vi "TrafficLight.vi"() -> ()   [LabVIEW 2020]
panel:
  in  "Car Speed":dbl(slide) scale=10.0..200.0
  out "E_3":bool
  out "E_2":bool
  out "E_1":bool
  out "W_3":bool
  out "W_2":bool
  out "W_1":bool
  out "S_3":bool
  out "S_2":bool
  out "S_1":bool
  out "N_3":bool
  out "N_2":bool
  out "N_1":bool
  in  "START":bool
  in  "EMERGENCY":bool
  in  "EW_Green Light Duration":dbl(slide) scale=5.0..30.0
  in  "NS_Green Light Duration":dbl(slide) scale=5.0..30.0
  in  "stop":bool
  out "W_R":bool
  out "W_Y":bool
  out "W_G":bool
  out "E_G":bool
  out "E_Y":bool
  out "E_R":bool
  out "S_G":bool
  out "S_Y":bool
  out "S_R":bool
  out "N_R":bool
  out "N_Y":bool
  out "N_G":bool
  # "Simulation Interface"
  # "Control Panel"
  # "North"
  # "West"
  # "East"
  # "South"
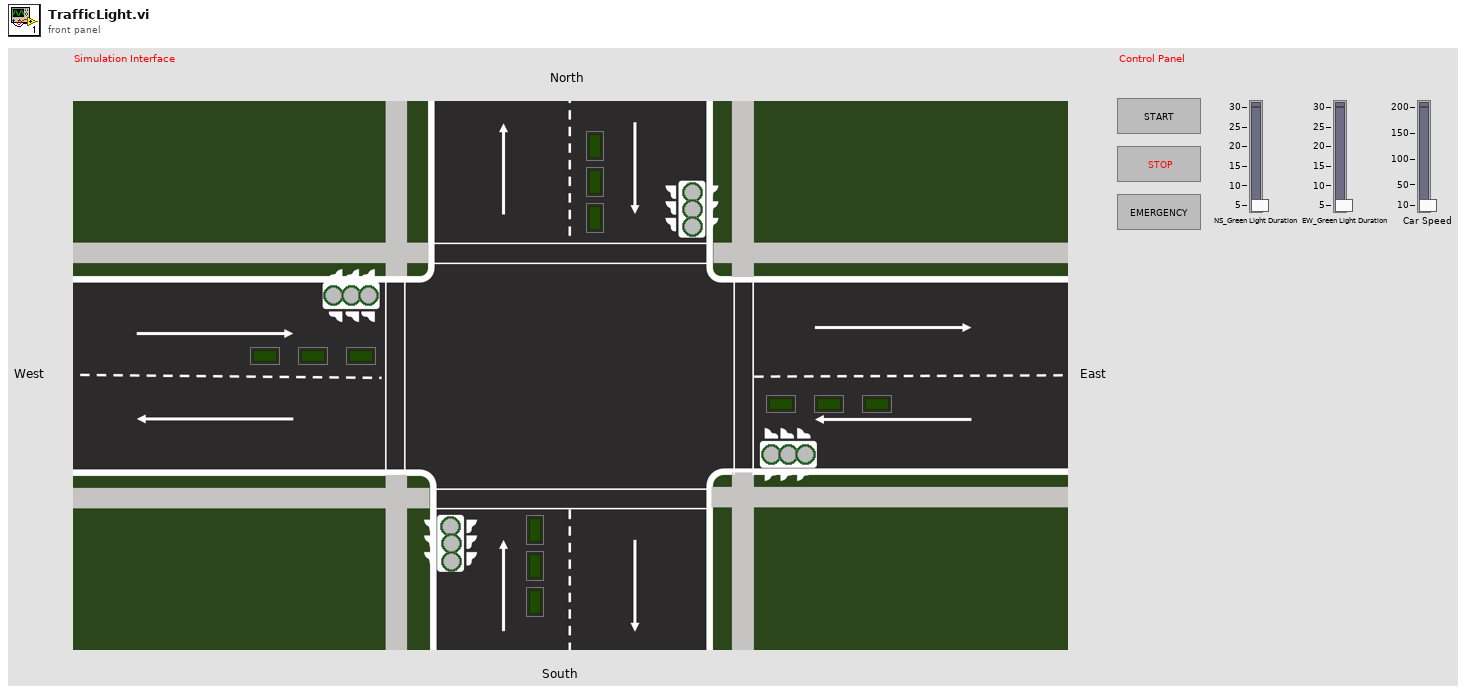
[diagram p1: front panel]
types:
  T1 = enum16{"Start", "Green", "Yellow", "Red", "Yellow'"}
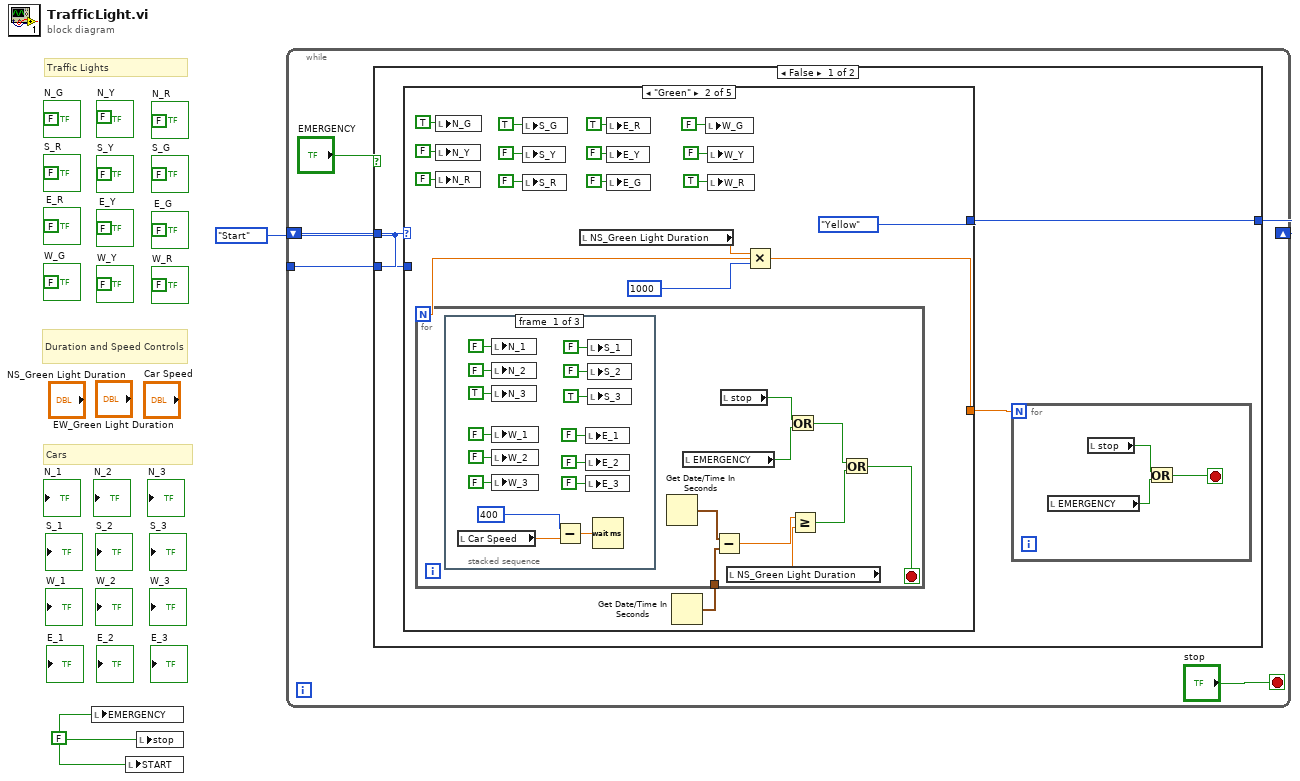
[diagram p0: block diagram]
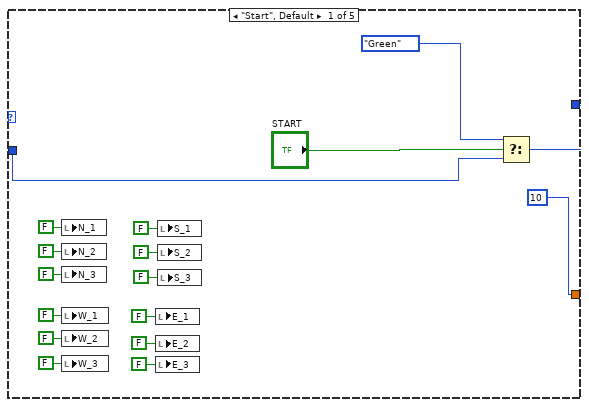
[diagram p2: hidden frame]
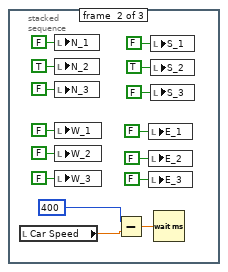
[diagram p3: hidden frame]
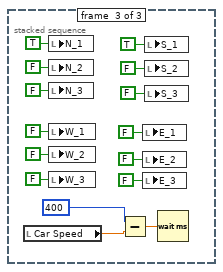
[diagram p4: hidden frame]
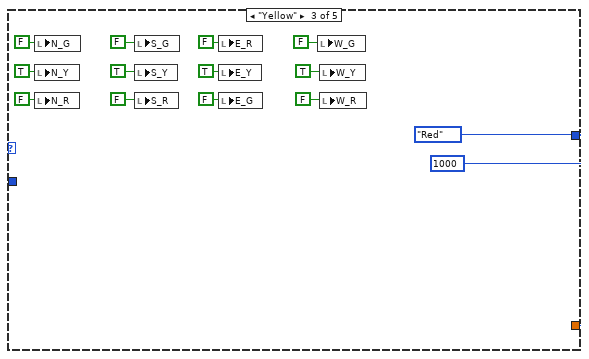
[diagram p5: hidden frame]
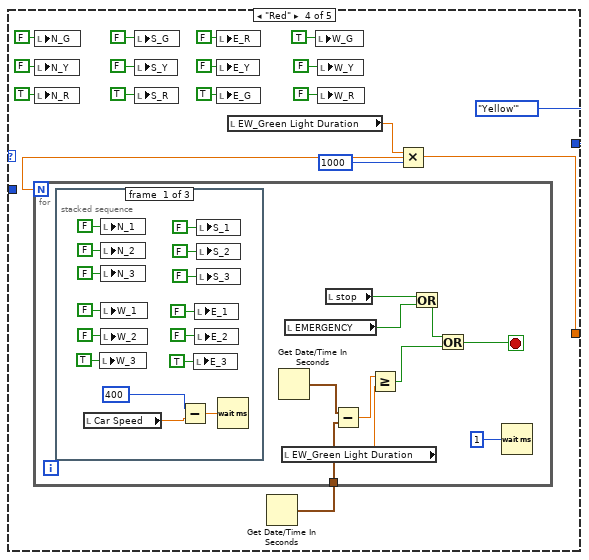
[diagram p6: hidden frame]
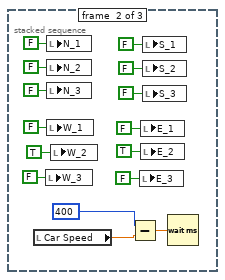
[diagram p7: hidden frame]
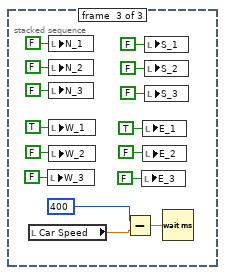
[diagram p8: hidden frame]
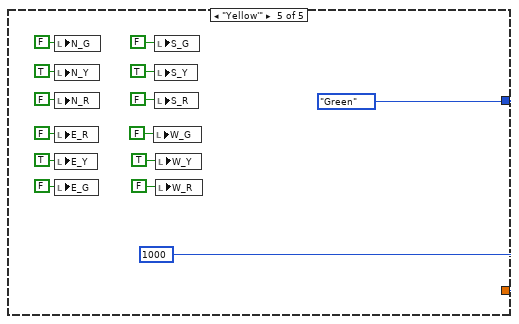
[diagram p9: hidden frame]
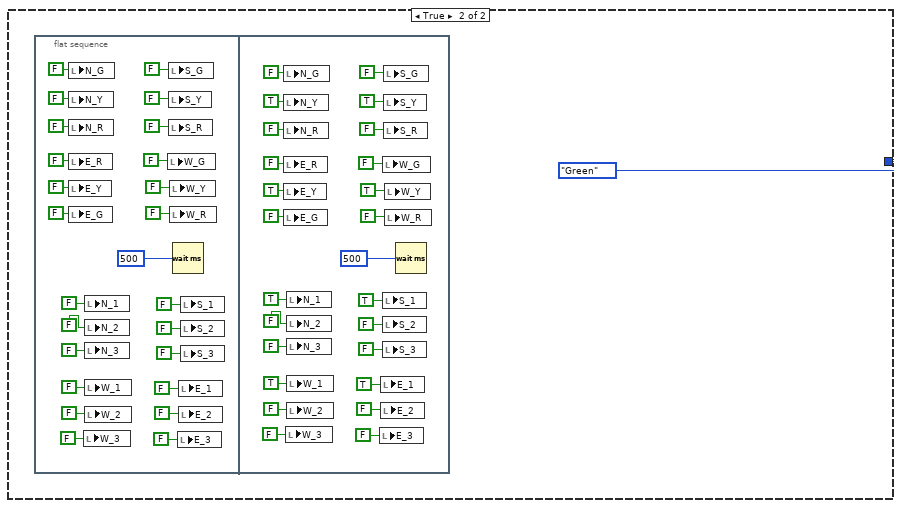
[diagram p10: hidden frame]
diagram:
  w1 = FALSE ("EMERGENCY")
  w2 = T1."Start"
  # "Cars"
  # "Duration and Speed Controls"
  # "Traffic Lights"
  n1 = local write "EMERGENCY"(w1) -> ()
  n2 = local write "START"(w1) -> ()
  n3 = local write "stop"(w1) -> ()
  n4 = while {
    shift-right: [w15] -> _
    shift-left: w2 -> [w17]
    tunnel: w2 -> [w16]
    stop <- "stop" stop-if-true
    n5 = case shown="False" "EMERGENCY" {
      tunnel: w17 -> [w23 _]
      tunnel: w16 -> [w22 _]
      tunnel: [w21 T1."Green"] -> w15
      frame False {
        n6 = case shown="\"Green\"" w23 {
          tunnel: w22 -> [w42 _ _ _ _]
          tunnel: [w40 T1."Yellow" T1."Red" T1."Yellow'" T1."Green"] -> w21
          tunnel: [10 w53 u32 1000 ("millisecond timer value") w130 u32 1000 ("millisecond timer value")] -> w20
          frame "Start", Default {
            (unwired) FALSE ("W_2")
            n7 = local write "N_1"(FALSE ("N_1")) -> ()
            n8 = local write "N_2"(FALSE ("N_2")) -> ()
            n9 = local write "N_3"(FALSE ("N_3")) -> ()
            n10 = local write "W_1"(FALSE ("W_1")) -> ()
            n11 = local write "W_2"(FALSE ("W_2")) -> ()
            n12 = local write "W_3"(FALSE ("W_3")) -> ()
            n13 = local write "E_1"(FALSE ("E_1")) -> ()
            n14 = local write "E_2"(FALSE ("E_2")) -> ()
            n15 = local write "E_3"(FALSE ("E_3")) -> ()
            n16 = local write "S_1"(FALSE ("S_1")) -> ()
            n17 = local write "S_2"(FALSE ("S_2")) -> ()
            n18 = local write "S_3"(FALSE ("S_3")) -> ()
            n19 = Select(t=T1."Green", s="START", f=w42) -> (s? t:f=w40:T1)
          }
          frame "Green" {
            n20 = local write "N_G"(TRUE ("N_G")) -> ()
            n21 = local write "N_Y"(FALSE ("N_Y")) -> ()
            n22 = local write "N_R"(FALSE ("N_R")) -> ()
            n23 = local write "S_G"(TRUE ("S_G")) -> ()
            n24 = local write "S_Y"(FALSE ("S_Y")) -> ()
            n25 = local write "S_R"(FALSE ("E_R")) -> ()
            n26 = local read "NS_Green Light Duration"() -> (w56:dbl)
            n27 = local write "E_R"(TRUE ("E_R")) -> ()
            n28 = local write "E_Y"(FALSE ("E_Y")) -> ()
            n29 = local write "E_G"(FALSE ("E_G")) -> ()
            n30 = Get Date/Time In Seconds() -> (seconds since 1Jan1904=w54:timestamp)
            n31 = local write "W_G"(FALSE ("W_G")) -> ()
            n32 = local write "W_Y"(FALSE ("W_Y")) -> ()
            n33 = local write "W_R"(TRUE ("W_R")) -> ()
            n34 = Multiply(x=w56, y=u32 1000 ("millisecond timer value")) -> (x*y=w53:dbl)
            n35 = for {
              N: w53 -> [_]
              tunnel: w54 -> [w68]
              stop <- w64 stop-if-true
              n36 = stacked-sequence {
                frame #0 {
                  (unwired) FALSE ("W_2")
                  n37 = local read "Car Speed"() -> (w70:dbl)
                  n38 = local write "N_1"(FALSE ("N_1")) -> ()
                  n39 = local write "N_2"(FALSE ("N_2")) -> ()
                  n40 = local write "N_3"(TRUE ("N_3")) -> ()
                  n41 = local write "W_1"(FALSE ("W_1")) -> ()
                  n42 = local write "W_2"(FALSE ("W_2")) -> ()
                  n43 = local write "W_3"(FALSE ("W_3")) -> ()
                  n44 = Subtract(x=u32 400 ("millisecond timer value"), y=w70) -> (x-y=w72:dbl)
                  n45 = local write "E_1"(FALSE ("E_1")) -> ()
                  n46 = local write "E_2"(FALSE ("E_2")) -> ()
                  n47 = local write "E_3"(FALSE ("E_3")) -> ()
                  n48 = local write "S_1"(FALSE ("S_1")) -> ()
                  n49 = local write "S_2"(FALSE ("S_2")) -> ()
                  n50 = local write "S_3"(TRUE ("S_3")) -> ()
                  n51 = Wait (ms)(milliseconds to wait=w72) -> ()  [unwired: 1 out]
                }
                frame #1 {
                  (unwired) FALSE ("W_2")
                  n52 = local read "Car Speed"() -> (w87:dbl)
                  n53 = local write "N_1"(FALSE ("N_1")) -> ()
                  n54 = local write "N_2"(TRUE ("N_2")) -> ()
                  n55 = local write "N_3"(FALSE ("N_3")) -> ()
                  n56 = local write "W_1"(FALSE ("W_1")) -> ()
                  n57 = local write "W_2"(FALSE ("W_2")) -> ()
                  n58 = local write "W_3"(FALSE ("W_3")) -> ()
                  n59 = Subtract(x=u32 400 ("millisecond timer value"), y=w87) -> (x-y=w85:dbl)
                  n60 = local write "E_1"(FALSE ("E_1")) -> ()
                  n61 = local write "E_2"(FALSE ("E_2")) -> ()
                  n62 = local write "E_3"(FALSE ("E_3")) -> ()
                  n63 = local write "S_1"(FALSE ("S_1")) -> ()
                  n64 = local write "S_2"(TRUE ("S_2")) -> ()
                  n65 = local write "S_3"(FALSE ("S_3")) -> ()
                  n66 = Wait (ms)(milliseconds to wait=w85) -> ()  [unwired: 1 out]
                }
                frame #2 {
                  (unwired) FALSE ("W_2")
                  n67 = local read "Car Speed"() -> (w100:dbl)
                  n68 = local write "N_1"(TRUE ("N_1")) -> ()
                  n69 = local write "N_2"(FALSE ("N_2")) -> ()
                  n70 = local write "N_3"(FALSE ("N_3")) -> ()
                  n71 = local write "W_1"(FALSE ("W_1")) -> ()
                  n72 = local write "W_2"(FALSE ("W_2")) -> ()
                  n73 = local write "W_3"(FALSE ("W_3")) -> ()
                  n74 = Subtract(x=u32 400 ("millisecond timer value"), y=w100) -> (x-y=w102:dbl)
                  n75 = local write "E_1"(FALSE ("E_1")) -> ()
                  n76 = local write "E_2"(FALSE ("E_2")) -> ()
                  n77 = local write "E_3"(FALSE ("E_3")) -> ()
                  n78 = local write "S_1"(TRUE ("S_1")) -> ()
                  n79 = local write "S_2"(FALSE ("S_2")) -> ()
                  n80 = local write "S_3"(FALSE ("S_3")) -> ()
                  n81 = Wait (ms)(milliseconds to wait=w102) -> ()  [unwired: 1 out]
                }
              }
              n82 = Get Date/Time In Seconds() -> (seconds since 1Jan1904=w69:timestamp)
              n83 = local read "EMERGENCY"() -> (w62:bool)
              n84 = Subtract(x=w69, y=w68) -> (x-y=w67:dbl)
              n85 = local read "stop"() -> (w63:bool)
              n86 = local read "NS_Green Light Duration"() -> (w66:dbl)
              n87 = Or(x=w63, y=w62) -> (x .or. y?=w61:bool)
              n88 = Greater Or Equal?(x=w67, y=w66) -> (x >= y?=w65:bool)
              n89 = Or(x=w61, y=w65) -> (x .or. y?=w64:bool)
            }
          }
          frame "Yellow" {
            n90 = local write "N_G"(FALSE ("N_G")) -> ()
            n91 = local write "N_Y"(TRUE ("N_Y")) -> ()
            n92 = local write "N_R"(FALSE ("N_R")) -> ()
            n93 = local write "S_G"(FALSE ("S_G")) -> ()
            n94 = local write "S_Y"(TRUE ("S_Y")) -> ()
            n95 = local write "S_R"(FALSE ("E_R")) -> ()
            n96 = local write "E_R"(FALSE ("E_R")) -> ()
            n97 = local write "E_Y"(TRUE ("E_Y")) -> ()
            n98 = local write "E_G"(FALSE ("E_G")) -> ()
            n99 = local write "W_G"(FALSE ("W_G")) -> ()
            n100 = local write "W_Y"(TRUE ("W_Y")) -> ()
            n101 = local write "W_R"(FALSE ("W_R")) -> ()
          }
          frame "Red" {
            n102 = local write "N_G"(FALSE ("N_G")) -> ()
            n103 = local write "N_Y"(FALSE ("N_Y")) -> ()
            n104 = local write "N_R"(TRUE ("N_R")) -> ()
            n105 = local write "S_G"(FALSE ("S_G")) -> ()
            n106 = local write "S_Y"(FALSE ("S_Y")) -> ()
            n107 = local write "S_R"(TRUE ("E_R")) -> ()
            n108 = local write "E_R"(FALSE ("E_R")) -> ()
            n109 = local write "E_Y"(FALSE ("E_Y")) -> ()
            n110 = local write "E_G"(TRUE ("E_G")) -> ()
            n111 = local read "EW_Green Light Duration"() -> (w131:dbl)
            n112 = Get Date/Time In Seconds() -> (seconds since 1Jan1904=w129:timestamp)
            n113 = local write "W_G"(TRUE ("W_G")) -> ()
            n114 = local write "W_Y"(FALSE ("W_Y")) -> ()
            n115 = local write "W_R"(FALSE ("W_R")) -> ()
            n116 = Multiply(x=w131, y=1000) -> (x*y=w130:dbl)
            n117 = for {
              N: w130 -> [_]
              tunnel: w129 -> [w153]
              stop <- w146 stop-if-true
              n118 = stacked-sequence {
                frame #0 {
                  (unwired) FALSE ("W_2")
                  n119 = local read "Car Speed"() -> (w156:dbl)
                  n120 = local write "W_3"(TRUE ("W_3")) -> ()
                  n121 = local write "N_1"(FALSE ("N_1")) -> ()
                  n122 = local write "N_2"(FALSE ("N_2")) -> ()
                  n123 = local write "N_3"(FALSE ("N_3")) -> ()
                  n124 = local write "W_1"(FALSE ("W_1")) -> ()
                  n125 = local write "W_2"(FALSE ("W_2")) -> ()
                  n126 = Subtract(x=u32 400 ("millisecond timer value"), y=w156) -> (x-y=w158:dbl)
                  n127 = local write "E_3"(TRUE ("E_3")) -> ()
                  n128 = local write "E_1"(FALSE ("E_1")) -> ()
                  n129 = local write "E_2"(FALSE ("E_2")) -> ()
                  n130 = local write "S_1"(FALSE ("S_1")) -> ()
                  n131 = local write "S_2"(FALSE ("S_2")) -> ()
                  n132 = local write "S_3"(FALSE ("S_3")) -> ()
                  n133 = Wait (ms)(milliseconds to wait=w158) -> ()  [unwired: 1 out]
                }
                frame #1 {
                  n134 = local read "Car Speed"() -> (w175:dbl)
                  n135 = local write "W_3"(FALSE ("W_3")) -> ()
                  n136 = local write "N_1"(FALSE ("N_1")) -> ()
                  n137 = local write "N_2"(FALSE ("N_2")) -> ()
                  n138 = local write "N_3"(FALSE ("N_3")) -> ()
                  n139 = local write "W_1"(FALSE ("W_1")) -> ()
                  n140 = local write "W_2"(TRUE ("W_2")) -> ()
                  n141 = Subtract(x=u32 400 ("millisecond timer value"), y=w175) -> (x-y=w173:dbl)
                  n142 = local write "E_3"(FALSE ("E_3")) -> ()
                  n143 = local write "E_1"(FALSE ("E_1")) -> ()
                  n144 = local write "E_2"(TRUE ("E_2")) -> ()
                  n145 = local write "S_1"(FALSE ("S_1")) -> ()
                  n146 = local write "S_2"(FALSE ("S_2")) -> ()
                  n147 = local write "S_3"(FALSE ("S_3")) -> ()
                  n148 = Wait (ms)(milliseconds to wait=w173) -> ()  [unwired: 1 out]
                }
                frame #2 {
                  (unwired) FALSE ("W_2")
                  n149 = local read "Car Speed"() -> (w186:dbl)
                  n150 = local write "W_3"(FALSE ("W_3")) -> ()
                  n151 = local write "N_1"(FALSE ("N_1")) -> ()
                  n152 = local write "N_2"(FALSE ("N_2")) -> ()
                  n153 = local write "N_3"(FALSE ("N_3")) -> ()
                  n154 = local write "W_1"(TRUE ("W_1")) -> ()
                  n155 = local write "W_2"(FALSE ("W_2")) -> ()
                  n156 = Subtract(x=u32 400 ("millisecond timer value"), y=w186) -> (x-y=w188:dbl)
                  n157 = local write "E_3"(FALSE ("E_3")) -> ()
                  n158 = local write "E_1"(TRUE ("E_1")) -> ()
                  n159 = local write "E_2"(FALSE ("E_2")) -> ()
                  n160 = local write "S_1"(FALSE ("S_1")) -> ()
                  n161 = local write "S_2"(FALSE ("S_2")) -> ()
                  n162 = local write "S_3"(FALSE ("S_3")) -> ()
                  n163 = Wait (ms)(milliseconds to wait=w188) -> ()  [unwired: 1 out]
                }
              }
              n164 = Get Date/Time In Seconds() -> (seconds since 1Jan1904=w154:timestamp)
              n165 = local read "EW_Green Light Duration"() -> (w151:dbl)
              n166 = local read "EMERGENCY"() -> (w149:bool)
              n167 = local read "stop"() -> (w150:bool)
              n168 = Subtract(x=w154, y=w153) -> (x-y=w152:dbl)
              n169 = Greater Or Equal?(x=w152, y=w151) -> (x >= y?=w147:bool)
              n170 = Or(x=w150, y=w149) -> (x .or. y?=w148:bool)
              n171 = Or(x=w148, y=w147) -> (x .or. y?=w146:bool)
              n172 = Wait (ms)(milliseconds to wait=u32 1 ("millisecond timer value")) -> ()  [unwired: 1 out]
            }
          }
          frame "Yellow'" {
            n173 = local write "N_G"(FALSE ("N_G")) -> ()
            n174 = local write "N_Y"(TRUE ("N_Y")) -> ()
            n175 = local write "N_R"(FALSE ("N_R")) -> ()
            n176 = local write "E_R"(FALSE ("E_R")) -> ()
            n177 = local write "E_Y"(TRUE ("E_Y")) -> ()
            n178 = local write "E_G"(FALSE ("E_G")) -> ()
            n179 = local write "W_G"(FALSE ("W_G")) -> ()
            n180 = local write "S_G"(FALSE ("S_G")) -> ()
            n181 = local write "S_Y"(TRUE ("S_Y")) -> ()
            n182 = local write "S_R"(FALSE ("E_R")) -> ()
            n183 = local write "W_Y"(TRUE ("W_Y")) -> ()
            n184 = local write "W_R"(FALSE ("W_R")) -> ()
          }
        }
        n185 = for {
          N: w20 -> [_]
          stop <- w24 stop-if-true
          n186 = local read "EMERGENCY"() -> (w25:bool)
          n187 = local read "stop"() -> (w26:bool)
          n188 = Or(x=w26, y=w25) -> (x .or. y?=w24:bool)
        }
      }
      frame True {
        n189 = flat-sequence {
          frame #0 {
            (unwired) FALSE ("W_2")
            n190 = local write "N_G"(FALSE ("N_G")) -> ()
            n191 = local write "N_Y"(FALSE ("N_Y")) -> ()
            n192 = local write "N_R"(FALSE ("N_R")) -> ()
            n193 = local write "E_R"(FALSE ("E_R")) -> ()
            n194 = local write "E_Y"(FALSE ("E_Y")) -> ()
            n195 = local write "E_G"(FALSE ("E_G")) -> ()
            n196 = local write "W_3"(FALSE ("W_3")) -> ()
            n197 = local write "N_1"(FALSE ("N_1")) -> ()
            n198 = local write "N_2"(FALSE ("N_2")) -> ()
            n199 = local write "N_3"(FALSE ("N_3")) -> ()
            n200 = local write "W_1"(FALSE ("W_1")) -> ()
            n201 = local write "W_2"(FALSE ("W_2")) -> ()
            n202 = local write "W_G"(FALSE ("W_G")) -> ()
            n203 = local write "S_G"(FALSE ("S_G")) -> ()
            n204 = local write "S_Y"(FALSE ("S_Y")) -> ()
            n205 = local write "S_R"(FALSE ("E_R")) -> ()
            n206 = local write "W_Y"(FALSE ("W_Y")) -> ()
            n207 = local write "W_R"(FALSE ("W_R")) -> ()
            n208 = Wait (ms)(milliseconds to wait=u32 500 ("millisecond timer value")) -> ()  [unwired: 1 out]
            n209 = local write "E_3"(FALSE ("E_3")) -> ()
            n210 = local write "E_1"(FALSE ("E_1")) -> ()
            n211 = local write "E_2"(FALSE ("E_2")) -> ()
            n212 = local write "S_1"(FALSE ("S_1")) -> ()
            n213 = local write "S_2"(FALSE ("S_2")) -> ()
            n214 = local write "S_3"(FALSE ("S_3")) -> ()
          }
          frame #1 {
            (unwired) FALSE ("W_2")
            n215 = local write "N_G"(FALSE ("N_G")) -> ()
            n216 = local write "N_Y"(TRUE ("N_Y")) -> ()
            n217 = local write "N_R"(FALSE ("N_R")) -> ()
            n218 = local write "E_R"(FALSE ("E_R")) -> ()
            n219 = local write "E_Y"(TRUE ("E_Y")) -> ()
            n220 = local write "E_G"(FALSE ("E_G")) -> ()
            n221 = local write "W_3"(FALSE ("W_3")) -> ()
            n222 = local write "N_1"(TRUE ("N_1")) -> ()
            n223 = local write "N_2"(FALSE ("N_2")) -> ()
            n224 = local write "N_3"(FALSE ("N_3")) -> ()
            n225 = local write "W_1"(TRUE ("W_1")) -> ()
            n226 = local write "W_2"(FALSE ("W_2")) -> ()
            n227 = local write "E_3"(FALSE ("E_3")) -> ()
            n228 = local write "E_1"(TRUE ("E_1")) -> ()
            n229 = local write "E_2"(FALSE ("E_2")) -> ()
            n230 = local write "W_G"(FALSE ("W_G")) -> ()
            n231 = local write "S_1"(TRUE ("S_1")) -> ()
            n232 = local write "S_2"(FALSE ("S_2")) -> ()
            n233 = local write "S_3"(FALSE ("S_3")) -> ()
            n234 = local write "S_G"(FALSE ("S_G")) -> ()
            n235 = local write "S_Y"(TRUE ("S_Y")) -> ()
            n236 = local write "S_R"(FALSE ("E_R")) -> ()
            n237 = local write "W_Y"(TRUE ("W_Y")) -> ()
            n238 = local write "W_R"(FALSE ("W_R")) -> ()
            n239 = Wait (ms)(milliseconds to wait=u32 500 ("millisecond timer value")) -> ()  [unwired: 1 out]
          }
        }
      }
    }
  }
  "N_G" <- FALSE ("N_G")
  "N_Y" <- FALSE ("N_Y")
  "N_R" <- FALSE ("N_R")
  "S_R" <- FALSE ("S_R")
  "S_Y" <- FALSE ("S_Y")
  "S_G" <- FALSE ("S_G")
  "E_R" <- FALSE ("E_R")
  "E_Y" <- FALSE ("E_Y")
  "E_G" <- FALSE ("E_G")
  "W_G" <- FALSE ("W_G")
  "W_Y" <- FALSE ("W_Y")
  "W_R" <- FALSE ("W_R")
